vi "Max_Array.vi"() -> ()   [LabVIEW 2024]
panel:
  out "Array":dbl[](array[numeric])
  out "max value":dbl
  out "max index(es)":i32
  in  "Numeric":i32
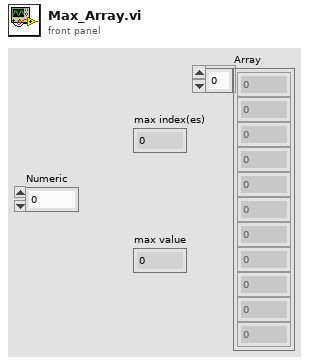
[diagram p1: front panel]
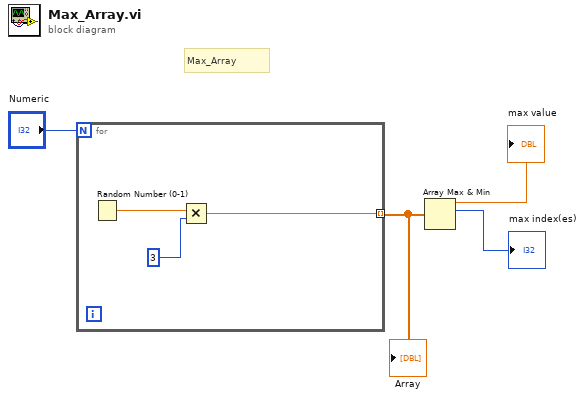
[diagram p0: block diagram]
diagram:
  # "Max_Array"
  n1 = for {
    N: "Numeric" -> [_]
    tunnel: [w5] -> w3 mode=indexing
    n2 = Random Number (0-1)() -> (number: 0 to 1=w7:dbl)
    n3 = Multiply(x=w7, y=3) -> (x*y=w5:dbl)
  }
  "Array" <- w3
  n4 = Array Max & Min(array=w3) -> (max value=→"max value":dbl, max index (indices)=→"max index(es)":i32)  [unwired: 2 out]
